vi "POO 1 - objet.vi"() -> ()   [LabVIEW 2020]
uses:
  Controller/Ctrl_ID.ctl
  ID/ID.lvclass
panel:
  out "Read ID 4":T1
  out "Read ID 3":T1
  in  "Write ID 2":T1
  out "Read ID 2":T1
  out "Read ID":T1
  in  "Write ID":T1
  # "Write"
  # "Read"
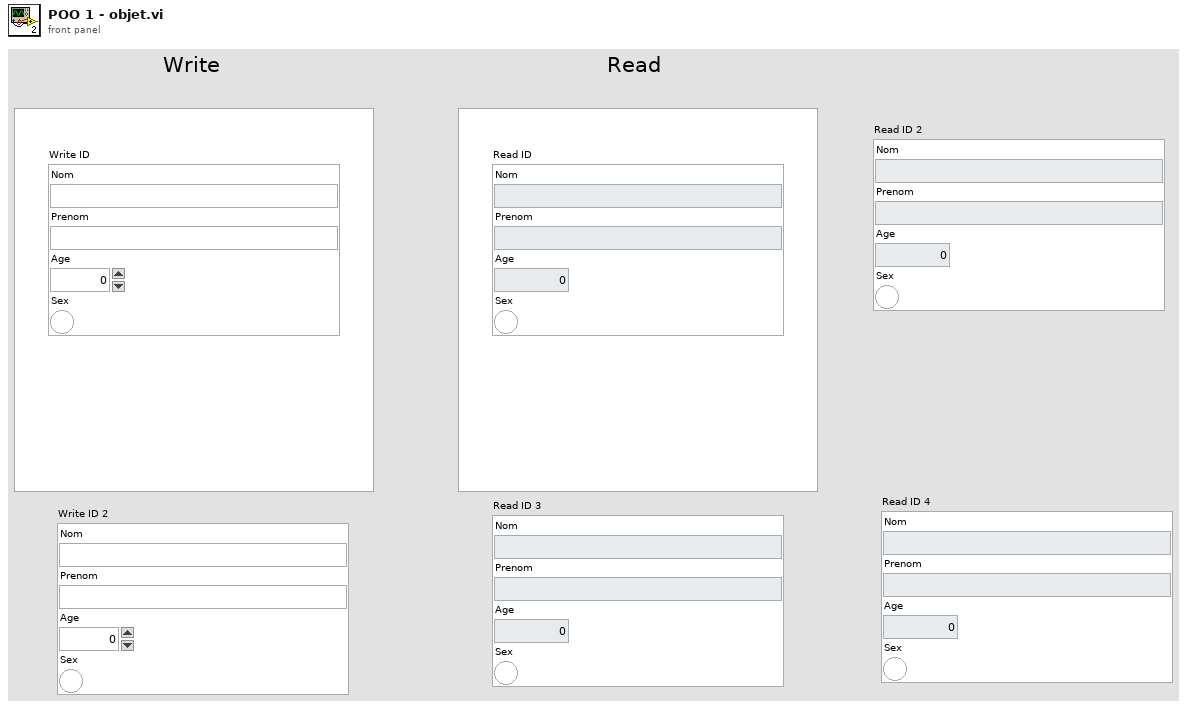
[diagram p1: front panel]
types:
  T1 = typedef "Ctrl_ID.ctl" = cluster{"Nom":string, "Prenom":string, "Age":u8, "Sex":bool}
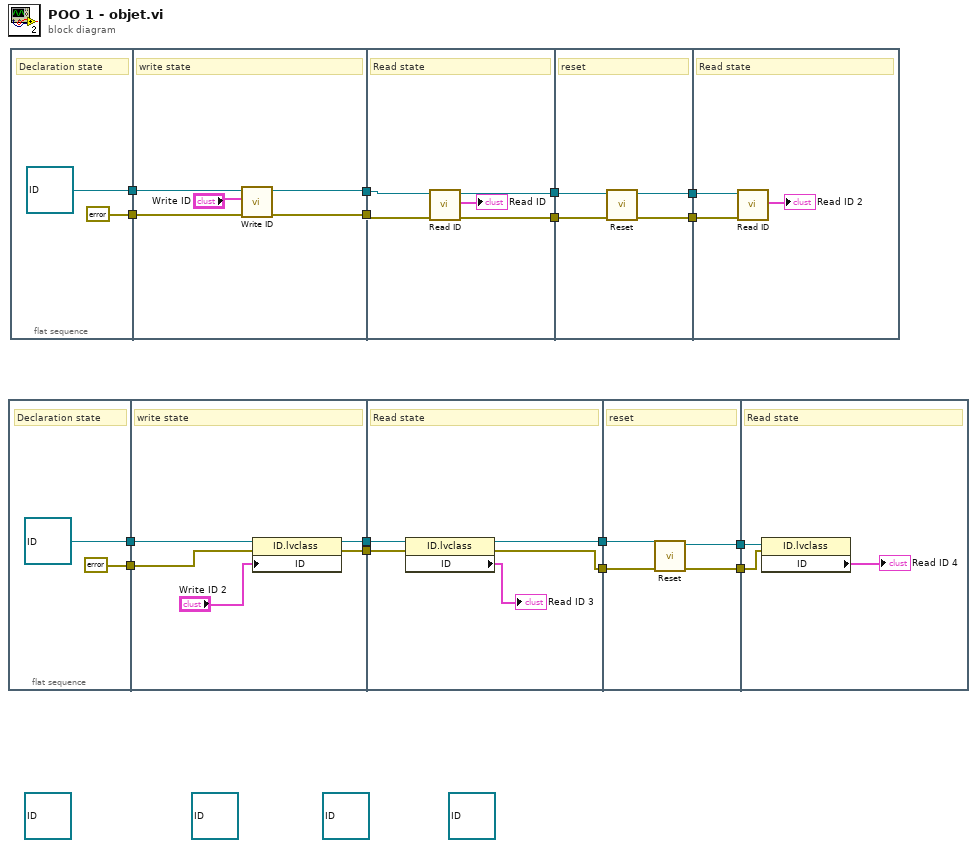
[diagram p0: block diagram]
diagram:
  (unwired) refnum<class "ID.lvclass"> refnum ("ID.lvclass")
  (unwired) refnum<class "ID.lvclass"> refnum ("ID.lvclass")
  (unwired) refnum<class "ID.lvclass"> refnum ("ID.lvclass")
  (unwired) refnum<class "ID.lvclass"> refnum ("ID.lvclass")
  n1 = flat-sequence {
    tunnel: [errorcluster {"status"=FALSE, "code"=0, "source"=""} ("error in (no error)")] -> w8
    tunnel: [refnum<class "ID.lvclass"> refnum ("ID.lvclass")] -> w7
    tunnel: w8 -> [w21]
    tunnel: w7 -> [w23]
    tunnel: [w20] -> w4
    tunnel: [w19] -> w3
    tunnel: w4 -> [w27]
    tunnel: w3 -> [w28]
    tunnel: [w25] -> w2
    tunnel: [w24] -> w1
    tunnel: [w32] -> w6
    tunnel: [w31] -> w5
    tunnel: w2 -> [w30]
    tunnel: w1 -> [w29]
    tunnel: w6 -> [w34]
    tunnel: w5 -> [w35]
    frame #0 {
      # "Declaration state"
    }
    frame #1 {
      # "write state"
      n2 = property class="ID.lvclass"(reference=w23, error in=w21, "ID"="Write ID 2") -> (reference out=w20:refnum<class "ID.lvclass">, error out=w19:errorcluster)
    }
    frame #2 {
      # "Read state"
      n3 = property class="ID.lvclass"(reference=w27, error in=w28) -> (reference out=w25:refnum<class "ID.lvclass">, error out=w24:errorcluster, "ID"=→"Read ID 3":T1)
    }
    frame #3 {
      # "reset"
      n4 = call-dynamic "Reset.vi"("error in (no error)"=w29, "ID in"=w30) -> ("error out"=w32:errorcluster, "ID out"=w31:refnum<class "ID.lvclass">)  [unwired: 8 in]
    }
    frame #4 {
      # "Read state"
      n5 = property class="ID.lvclass"(reference=w35, error in=w34) -> ("ID"=→"Read ID 4":T1)  [unwired: 2 out]
    }
  }
  n6 = flat-sequence {
    tunnel: [errorcluster {"status"=FALSE, "code"=0, "source"=""} ("error in (no error)")] -> w16
    tunnel: [refnum<class "ID.lvclass"> refnum ("ID.lvclass")] -> w15
    tunnel: w16 -> [w41]
    tunnel: w15 -> [w40]
    tunnel: [w42] -> w14
    tunnel: [w38] -> w13
    tunnel: w14 -> [w47]
    tunnel: w13 -> [w46]
    tunnel: [w44] -> w12
    tunnel: [w43] -> w11
    tunnel: w12 -> [w51]
    tunnel: w11 -> [w50]
    tunnel: [w49] -> w10
    tunnel: [w48] -> w9
    tunnel: w10 -> [w53]
    tunnel: w9 -> [w52]
    frame #0 {
      # "Declaration state"
    }
    frame #1 {
      # "write state"
      n7 = call-dynamic "Write ID.vi"("error in (no error)"=w41, "ID"="Write ID", "ID in"=w40) -> ("error out"=w42:errorcluster, "ID out"=w38:refnum<class "ID.lvclass">)  [unwired: 7 in]
    }
    frame #2 {
      # "Read state"
      n8 = call-dynamic "Read ID.vi"("error in (no error)"=w47, "ID in"=w46) -> ("error out"=w44:errorcluster, "ID"=→"Read ID":T1, "ID out"=w43:refnum<class "ID.lvclass">)  [unwired: 7 in]
    }
    frame #3 {
      # "reset"
      n9 = call-dynamic "Reset.vi"("error in (no error)"=w51, "ID in"=w50) -> ("error out"=w49:errorcluster, "ID out"=w48:refnum<class "ID.lvclass">)  [unwired: 8 in]
    }
    frame #4 {
      # "Read state"
      n10 = call-dynamic "Read ID.vi"("error in (no error)"=w53, "ID in"=w52) -> ("ID"=→"Read ID 2":T1)  [unwired: 7 in, 2 out]
    }
  }
